vi "CalculateCurvature.vi"(9 "Robot":T1 {"Angle" scale=0.0..360.0; "Point"."y" scale=-10.0..10.0; "Point"."x" scale=-10.0..10.0}, 10 "Lookahead":dbl, 11 "Point":cluster{"x":dbl, "y":dbl}) -> (3 "Curvature":dbl)   [LabVIEW 2020]
doc: "Calculates the curvature of the circle that gets the robot to the lookahead point, given lookahead distance, robot location/angle, and the lookahead point"
panel:
  out "output variable":dbl
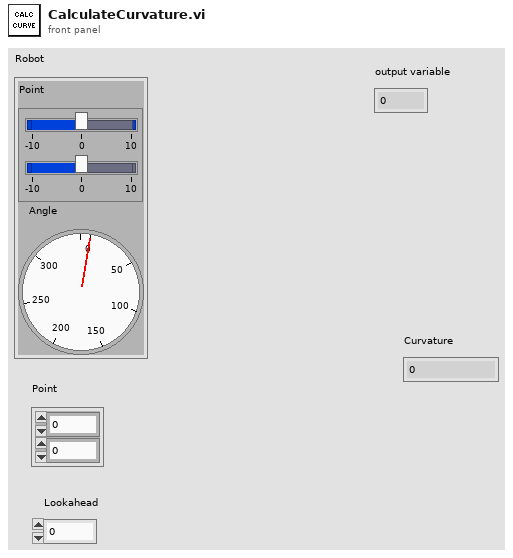
[diagram p1: front panel]
types:
  T1 = cluster{"Point":cluster{"x":dbl, "y":dbl}, "Angle":dbl}
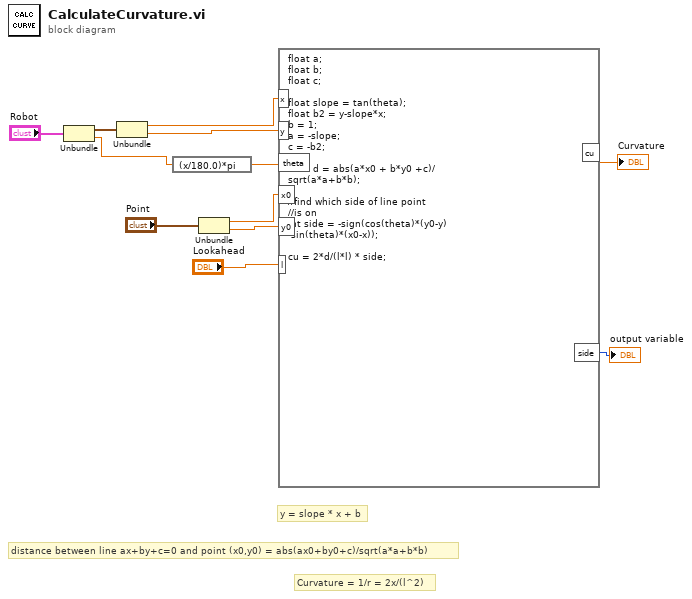
[diagram p0: block diagram]
diagram:
  # "Curvature = 1/r = 2x/(l^2)"
  # "y = slope * x + b"
  # "distance between line ax+by+c=0 and point (x0,y0) = abs(ax0+by0+c)/sqrt(a*a+b*b)"
  n1 = Unbundle("Robot") -> ("Point"=w11:cluster{"x":dbl, "y":dbl}, "Angle"=w1:dbl)
  n2 = Unbundle(w11) -> ("x"=w10:dbl, "y"=w9:dbl)
  n3 = expression code="(x/180.0)*pi" ("degrees to radians")(w1) -> (w8:dbl)
  n4 = Unbundle("Point") -> ("x"=w6:dbl, "y"=w5:dbl)
  n5 = formula code="float a;\nfloat b;\nfloat c;\n\nfloat slope = tan(theta);\nfloat b2 = y-slope*x;\nb = 1;\na = -slope;\nc = -b2;\n\nfloat d = abs(a*x0 + b*y0 +c)/\nsqrt(a*a+b*b);\n\n//find which side of line point\n//is on\nint side = -sign(cos(theta)*(y0-y)\n-sin(theta)*(x0-x));\n\ncu = 2*d/(l*l) * side;"("x"=w10, "y"=w9, "theta"=w8, "x0"=w6, "y0"=w5, "l"="Lookahead") -> ("cu"=→"Curvature":dbl, "side"=→"output variable":i32)
